vi "Write.vi"(8 "error in (no error)":errorcluster, 11 "Key in":refnum<class "Key.lvclass">) -> (0 "error out":errorcluster, 3 "Key out":refnum<class "Key.lvclass">)   [LabVIEW 2021, in "Library.lvlib" / "Key.lvclass"]
uses:
  Key.lvclass
  Key.lvclass/Key.ctl
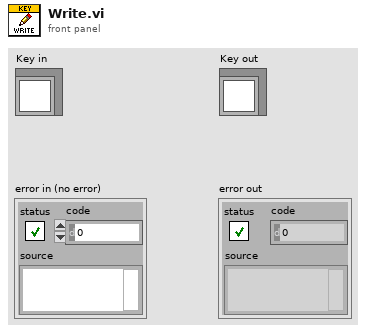
[diagram p1: front panel]
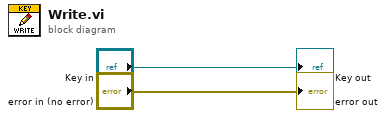
[diagram p0: block diagram]
diagram:
  "error out" <- "error in (no error)"
  "Key out" <- "Key in"
